vi "RunTillAbortTest.vi"() -> ()   [LabVIEW 2014]
panel:
  out "Start Acquisition Error Code":u32
  out "2":u32
  out "1":u32
  out "Numeric":i32
  in  "stop":bool
  out "4":u32
  out "Return from Get Acquisition":u32=20002
  out "Intensity Graph":i32[][](graph)
  out "3":u32
  out "Return from GetStatus":u32=73
  out "0":u32
  in  "vend":i32=512
  in  "vstart":i32=1
  in  "hend":i32=512
  in  "hstart":i32=1
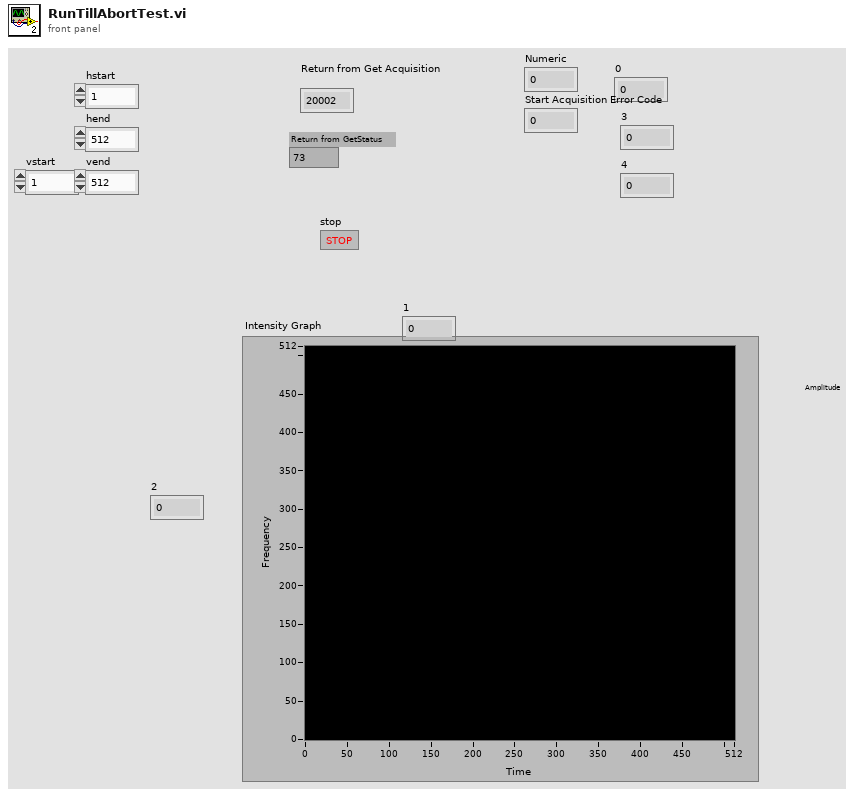
[diagram p1: front panel]
types:
  T1 = typedef "Error Code Enum typedef.ctl" = enum32{"N/A (0)", "DRV_ERROR_CODES", "DRV_SUCCESS", "DRV_VXDNOTINSTALLED", "DRV_ERROR_SCAN", "DRV_ERROR_CHECK_SUM", "DRV_ERROR_FILELOAD", "DRV_UNKNOWN_FUNC", "DRV_ERROR_VXD_INIT", "DRV_ERROR_ADDRESS", "DRV_ERROR_PAGELOCK", "DRV_ERROR_PAGEUNLOCK", "DRV_ERROR_BOARDTEST", "DRV_ERROR_ACK", "DRV_ERROR_UP_FIFO", "DRV_ERROR_PATTERN", "N/A (16)", "DRV_ACQUISITION_ERRORS", "DRV_ACQ_BUFFER", "DRV_ACQ_DOWNFIFO_FULL", "DRV_PROC_UNKONWN_INSTRUCTION", "DRV_ILLEGAL_OP_CODE", "DRV_KINETIC_TIME_NOT_MET", "DRV_ACCUM_TIME_NOT_MET", "DRV_NO_NEW_DATA", "N/A (25)", "DRV_SPOOLERROR", "N/A (27)", "N/A (28)", "N/A (29)", "N/A (30)", "N/A (31)", "N/A (32)", "DRV_TEMPERATURE_CODES", "DRV_TEMPERATURE_OFF", "DRV_TEMPERATURE_NOT_STABILIZED", "DRV_TEMPERATURE_STABILIZED", "DRV_TEMPERATURE_NOT_REACHED", "DRV_TEMPERATURE_OUT_RANGE", "DRV_TEMPERATURE_NOT_SUPPORTED", "DRV_TEMPERATURE_DRIFT", "N/A (41)", "N/A (42)", "N/A (43)", "N/A (44)", "N/A (45)", "N/A (46)", "N/A (47)", "N/A (48)", "DRV_GENERAL_ERRORS", "DRV_INVALID_AUX", "DRV_COF_NOTLOADED", "DRV_FPGAPROG", "DRV_FLEXERROR", "DRV_GPIBERROR", "N/A (55)", "N/A (56)", "N/A (57)", "N/A (58)", "N/A (59)", "N/A (60)", "N/A (61)", "N/A (62)", "N/A (63)", "DRV_DATATYPE", "DRV_DRIVER_ERRORS", "DRV_P1INVALID", "DRV_P2INVALID", "DRV_P3INVALID", "DRV_P4INVALID", "DRV_INIERROR", "DRV_COFERROR", "DRV_ACQUIRING", "DRV_IDLE", "DRV_TEMPCYCLE", "DRV_NOT_INITIALIZED", "DRV_P5INVALID", "DRV_P6INVALID", "DRV_INVALID_MODE", "DRV_INVALID_FILTER", "DRV_I2CERRORS", "DRV_I2CDEVNOTFOUND", "DRV_I2CTIMEOUT", "DRV_P7INVALID", "N/A (84)", "N/A (85)", "N/A (86)", "N/A (87)", "N/A (88)", "N/A (89)", "DRV_IOCERROR", "DRV_VRMVERSIONERROR"}
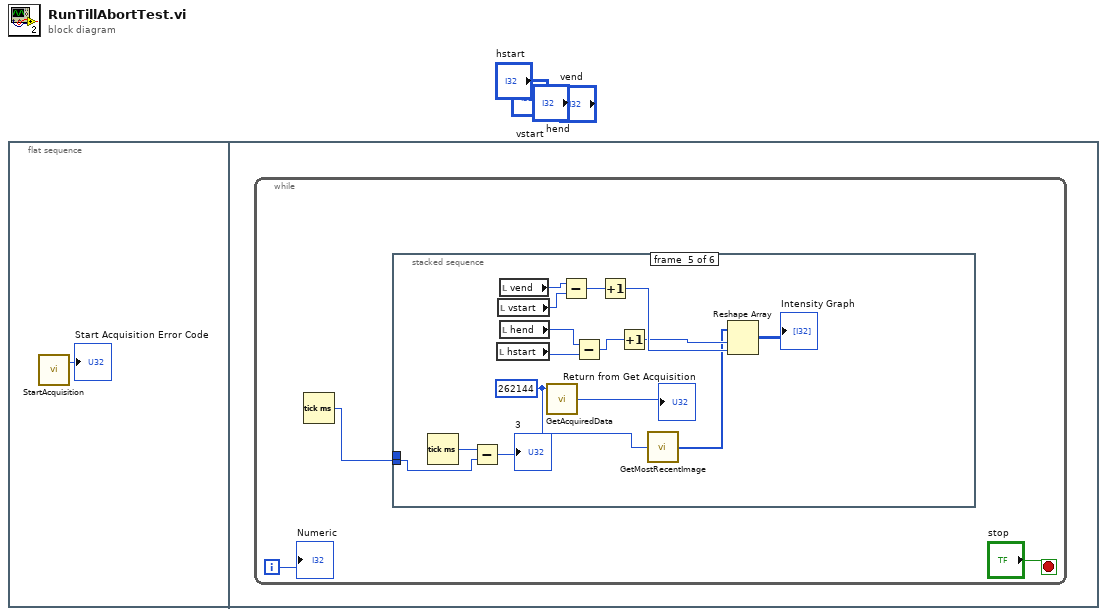
[diagram p0: block diagram]
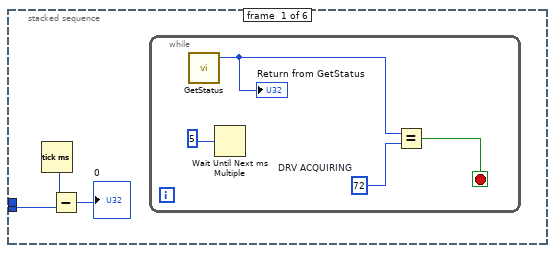
[diagram p2: hidden frame]
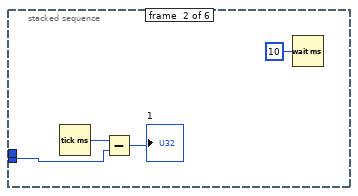
[diagram p3: hidden frame]
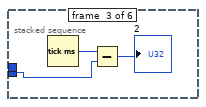
[diagram p4: hidden frame]
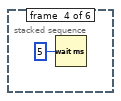
[diagram p5: hidden frame]
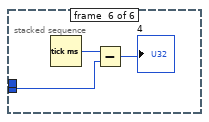
[diagram p6: hidden frame]
diagram:
  n1 = flat-sequence {
    frame #0 {
      n2 = call "StartAcquisition.vi"() -> ("DLL error code"=→"Start Acquisition Error Code":u32)  [unwired: 2 in, 1 out]
    }
    frame #1 {
      n3 = while {
        i -> [w2]
        stop <- "stop" stop-if-true
        n4 = Tick Count (ms)() -> (millisecond timer value=w4:u32)
        n5 = stacked-sequence {
          tunnel: w4 -> [w5 w12 w16 _ w22 w35]
          tunnel: [_ _ w16 _ _ _] -> _
          frame #0 {
            n6 = Tick Count (ms)() -> (millisecond timer value=w7:u32)
            n7 = Subtract(x=w7, y=w5) -> (x-y=→"0":u32)
            n8 = while {
              stop <- w10 stop-if-true
              w9 = u16 72  # DRV ACQUIRING
              n9 = call "GetStatus.vi"() -> ("status"=w8:T1)  [unwired: 3 in, 2 out]
              "Return from GetStatus" <- w8
              n10 = Wait Until Next ms Multiple(millisecond multiple=u32 5) -> ()  [unwired: 1 out]
              n11 = Equal?(x=w8, y=w9) -> (x = y?=w10:bool)
            }
          }
          frame #1 {
            n12 = Tick Count (ms)() -> (millisecond timer value=w13:u32)
            n13 = Subtract(x=w13, y=w12) -> (x-y=→"1":u32)
            n14 = Wait (ms)(milliseconds to wait=u32 10) -> ()  [unwired: 1 out]
          }
          frame #2 {
            n15 = Tick Count (ms)() -> (millisecond timer value=w18:u32)
            n16 = Subtract(x=w18, y=w16) -> (x-y=→"2":u32)
          }
          frame #3 {
            n17 = Wait (ms)(milliseconds to wait=u32 5) -> ()  [unwired: 1 out]
          }
          frame #4 {
            w21 = u32 262144 ("size")
            n18 = Tick Count (ms)() -> (millisecond timer value=w24:u32)
            n19 = Subtract(x=w24, y=w22) -> (x-y=→"3":u32)
            n20 = local read "hstart"() -> (w30:i32)
            n21 = local read "vstart"() -> (w32:i32)
            n22 = local read "vend"() -> (w33:i32)
            n23 = local read "hend"() -> (w31:i32)
            n24 = call "GetAcquiredData.vi"("size"=w21) -> ("DLL error code"=→"Return from Get Acquisition":u32)  [unwired: 2 in, 2 out]
            n25 = Subtract(x=w33, y=w32) -> (x-y=w29:i32)
            n26 = Subtract(x=w31, y=w30) -> (x-y=w28:i32)
            n27 = Increment(x=w29) -> (x+1=w26:i32)
            n28 = Increment(x=w28) -> (x+1=w25:i32)
            n29 = call "GetMostRecentImage.vi"("size"=w21) -> ("array"=w20:i32[])  [unwired: 2 in, 2 out]
            n30 = Reshape Array(w20, w25, w26) -> (→"Intensity Graph":i32[][])
          }
          frame #5 {
            n31 = Tick Count (ms)() -> (millisecond timer value=w37:u32)
            n32 = Subtract(x=w37, y=w35) -> (x-y=→"4":u32)
          }
        }
        "Numeric" <- w2
      }
    }
  }
